vi "Power Accuracy Update Points Listbox.vi"(6 "Colors":cluster{"Pass":u32, "Fail":u32, "Nop":u32}={"Pass"=6618880, "Fail"=16711680, "Nop"=16777226}, 7 "State (Pass/Fail)":enum16{"Reset", "In Progress", "Pass/Fail"}(ring), 8 "error in (no error)":errorcluster, 9 "Pass/Fail":bool[](array[boolean]), 10 "Stimulus":T1={"Power Start"=38, "Power Stop"=46, "Frequency Type"=enum."Band Edges", "Frequency Points"=[], "TX 1 Frequency (MHz)"={"Min"=0.0, "Max"=0.0}, "TX 2 Frequency (MHz)"={"Min"=0.0, "Max"=0.0}, "RX Frequency (MHz)"={"Min"=0.0, "Max"=0.0}, "Pad Model Number"="", "Pad Serial Number"="", "Pad Values"=[]}, 11 "Points Measured":refnum<vi>) -> (0 "error out":errorcluster, 3 "Points Measured":refnum<vi>)   [LabVIEW 2011]
uses:
  TypeDefs/Power Accuracy Stimulus Parameters.ctl
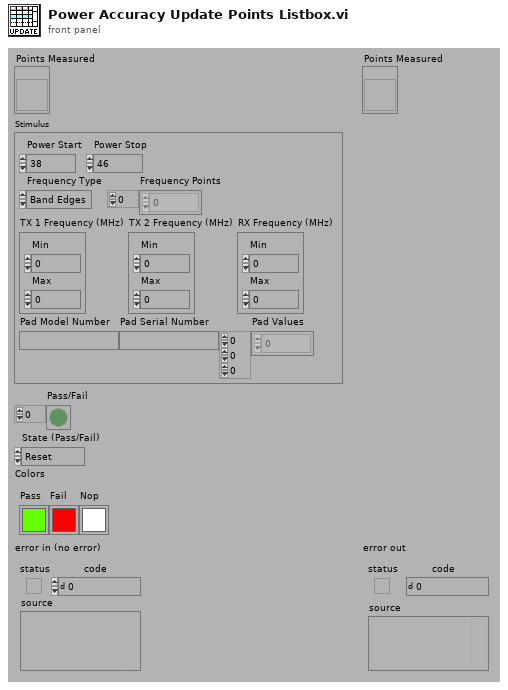
[diagram p1: front panel]
types:
  T1 = typedef "Power Accuracy Stimulus Parameters.ctl" = cluster{"Power Start":i32, "Power Stop":i32, "Frequency Type":enum16{"Band Edges", "Custom"}, "Frequency Points":dbl[], "TX 1 Frequency (MHz)":cluster{"Min":dbl, "Max":dbl}, "TX 2 Frequency (MHz)":cluster{"Min":dbl, "Max":dbl}, "RX Frequency (MHz)":cluster{"Min":dbl, "Max":dbl}, "Pad Model Number":string, "Pad Serial Number":string, "Pad Values":dbl[][][]}
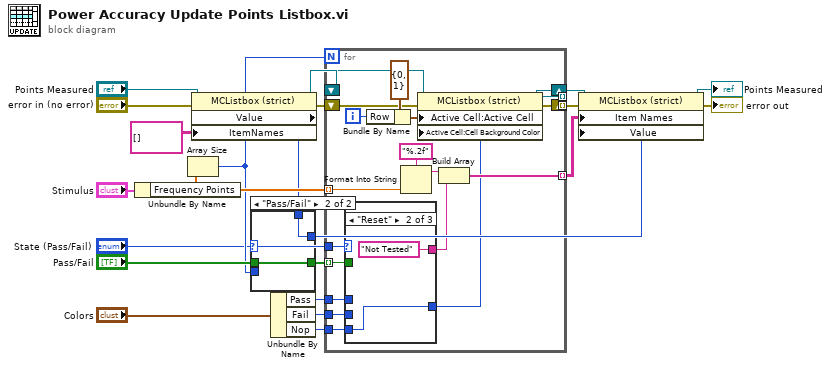
[diagram p0: block diagram]
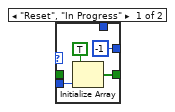
[diagram p2: hidden frame]
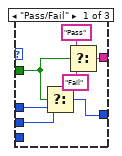
[diagram p3: hidden frame]
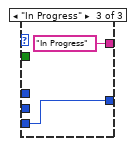
[diagram p4: hidden frame]
diagram:
  n1 = Unbundle By Name("Stimulus") -> ("Frequency Points"=w15:dbl[])
  n2 = Array Size(array=w15) -> (size(s)=w14:i32)
  n3 = property class="MCListbox (strict)"(reference="Points Measured", error in="error in (no error)", "ItemNames"=string[][] [] ("Item Names")) -> (reference out=w10:refnum<vi>, error out=w9:errorcluster, "Value"=w1:i32)
  n4 = case shown="\"Pass/Fail\"" "State (Pass/Fail)" {
    tunnel: [w25 w28] -> w18
    tunnel: "Pass/Fail" -> [_ w28]
    tunnel: w14 -> [w24 _]
    tunnel: [-1 ("Value") w27] -> w2
    tunnel: w1 -> [_ w27]
    frame "Reset", "In Progress" {
      n5 = Initialize Array(TRUE, w24) -> (w25:bool[])
    }
    frame "Pass/Fail" {
    }
  }
  n6 = Unbundle By Name("Colors") -> ("Pass"=w21:u32, "Fail"=w20:u32, "Nop"=w19:u32)
  n7 = for {
    N: w14 -> [_]
    tunnel: w21 -> [w37]
    tunnel: w20 -> [w36]
    shift-right: [w29] -> w7
    shift-left: w9 -> [w43]
    tunnel: [w42] -> w5 mode=indexing
    tunnel: w18 -> [w35] mode=indexing
    tunnel: w19 -> [w33]
    tunnel: "State (Pass/Fail)" -> [w34]
    tunnel: w15 -> [w31] mode=indexing
    shift-right: [w30] -> w6
    shift-left: w10 -> [w44]
    tunnel: [w30] -> _ mode=indexing
    tunnel: [w29] -> _ mode=indexing
    i -> [w32]
    n8 = case shown="\"Reset\"" w34 {
      tunnel: [w49 "Not Tested" "In Progress"] -> w39
      tunnel: [w53 w54 w56] -> w38
      tunnel: w37 -> [w52 _ _]
      tunnel: w36 -> [w51 _ _]
      tunnel: w35 -> [w50 _ _]
      tunnel: w33 -> [_ w54 w56]
      frame "Pass/Fail" {
        n9 = Select(t=w52, s=w50, f=w51) -> (s? t:f=w53:u32)
        n10 = Select(t="Pass" ("format string"), s=w50, f="Fail" ("format string")) -> (s? t:f=w49:string)
      }
      frame "Reset" {
      }
      frame "In Progress" {
      }
    }
    n11 = Bundle By Name(cluster=cluster{"Row":i32, "Column":i32} {"Row"=0, "Column"=1} ("Active Cell"), "Row"=w32) -> (w45:cluster{"Row":i32, "Column":i32})
    n12 = Format Into String(format string="%.2f", w31) -> (resulting string=w40:string)  [unwired: 2 in, 1 out]
    n13 = property class="MCListbox (strict)"(reference=w44, error in=w43, "Active Cell:Active Cell"=w45, "Active Cell:Cell Background Color"=w38) -> (reference out=w30:refnum<vi>, error out=w29:errorcluster)
    n14 = Build Array(w40, w39) -> (w42:string[])
  }
  n15 = property class="MCListbox (strict)"(reference=w6, error in=w7, "Item Names"=w5, "Value"=w2) -> (reference out=→"Points Measured":refnum<vi>, error out=→"error out":errorcluster)
